vi "function1.vi"   [LabVIEW 2016, in "Test2.lvrbt"]
uses:
  Test2.lvrbt
  <vilib>/NXT/Hardware/Plugins/Tetrix DC Motor/TetrixDCMotorAddress.ctl
  <vilib>/NXT/Block Support/NXT_InputPort.ctl
  <vilib>/NXT/NXTIO Xnodes/NXTIONodeSubVIs/TETRIX IO Move DC Motors.vi
  <vilib>/NXT/Dual Mode Library/Waits/Wait_EV3_Ultrasonic_Centimeter_Closer.vi
  <vilib>/NXT/NXTIO Xnodes/NXTIONodeSubVIs/TETRIX IO Stop DC Motors.vi
  <vilib>/NXT/Dual Mode Library/Waits/Wait_Num.vi
  <vilib>/NXT/Dual Mode Library/Waits/Wait_EV3_Ultrasonic_Centimeters_Further.vi
  <vilib>/NXT/Subs/LVHSConnector.ctl
  <vilib>/NXT/NXTIO Xnodes/AddressXNode/NXTIOAddress.xnode
  <vilib>/NXT/NXTIO Xnodes/NXTIOXNode/NXTIO.xnode
  <vilib>/NXT/LegoClasses/BrickReference/BrickReference.lvclass
types:
  T1 = typedef "TetrixDCMotorAddress.ctl" = i32
  T2 = typedef "LVHSConnector.ctl" = refnum<class "BrickReference.lvclass">
  T3 = typedef "NXT_InputPort.ctl" = u32
  T4 = cluster{"TetrixDCMotor":T1, "TetrixDCMotor 2":T1}
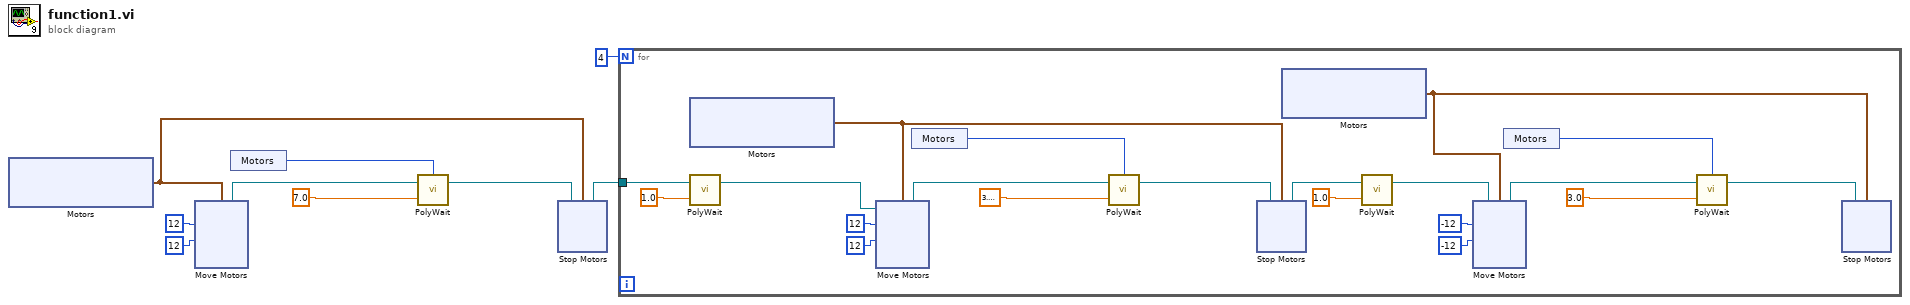
[diagram p0: block diagram]
diagram:
  n1 = xnode "Motors"() -> ("Motor"=w3:cluster{"TetrixDCMotor":T1, "TetrixDCMotor":T1})
  n2 = xnode "Move Motors"("Power/Speed 2"=i8 12, "Power/Speed 1"=i8 12, "Motors"=w3) -> ("NXT/EV3"=w6:T2)  [unwired: 1 in]
  n3 = xnode "Motors"() -> ("Sensor"=w2:T3)
  n4 = call-poly <vilib>:"PolyWait.vi"("Centimeters (40)"=sgl 7.0, "NXT/EV3"=w6, "Port (Port 1)"=w2) -> ("NXT/EV3"=w4:T2)  [unwired: 1 in]
  n5 = xnode "Stop Motors"("Motors"=w3, "NXT/EV3"=w4) -> ("NXT/EV3"=w1:T2)
  n6 = for {
    N: 4 -> [_]
    tunnel: w1 -> [w10]
    n7 = xnode "Motors"() -> ("Motor"=w24:cluster{"TetrixDCMotor":T1, "TetrixDCMotor":T1})
    n8 = call-poly <vilib>:"PolyWait.vi"("Time (1 sec)"=sgl 1.0, "NXT/EV3"=w10) -> ("NXT/EV3"=w13:T2)  [unwired: 2 in]
    n9 = xnode "Move Motors"("Power/Speed 2"=i8 12, "Power/Speed 1"=i8 12, "Motors"=w24, "NXT/EV3"=w13) -> ("NXT/EV3"=w27:T2)
    n10 = xnode "Motors"() -> ("Sensor"=w12:T3)
    n11 = call-poly <vilib>:"PolyWait.vi"("Centimeters (40)"=sgl 3.2, "NXT/EV3"=w27, "Port (Port 1)"=w12) -> ("NXT/EV3"=w25:T2)  [unwired: 1 in]
    n12 = xnode "Stop Motors"("Motors"=w24, "NXT/EV3"=w25) -> ("NXT/EV3"=w22:T2)
    n13 = xnode "Motors"() -> ("Motor"=w15:cluster{"TetrixDCMotor":T1, "TetrixDCMotor":T1})
    n14 = call-poly <vilib>:"PolyWait.vi"("Time (1 sec)"=sgl 1.0, "NXT/EV3"=w22) -> ("NXT/EV3"=w21:T2)  [unwired: 2 in]
    n15 = xnode "Move Motors"("Power/Speed 2"=i8 -12, "Power/Speed 1"=i8 -12, "Motors"=w15, "NXT/EV3"=w21) -> ("NXT/EV3"=w18:T2)
    n16 = xnode "Motors"() -> ("Sensor"=w11:T3)
    n17 = call-poly <vilib>:"PolyWait.vi"("Centimeters (50)"=sgl 3.0, "NXT/EV3"=w18, "Port (Port 1)"=w11) -> ("NXT/EV3"=w16:T2)  [unwired: 1 in]
    n18 = xnode "Stop Motors"("Motors"=w15, "NXT/EV3"=w16) -> ()  [unwired: 1 out]
  }
